vi "Get Cooler Status.vi"(8 "error in (no error)":errorcluster, 11 "Detector in":refnum<class "Detector.lvclass">) -> (0 "error out":errorcluster, 2 "Cooler status":bool, 3 "Detector out":refnum<class "Detector.lvclass">)   [LabVIEW 2015, in "Detector.lvclass"]
uses:
  Detector.lvclass
  GeneralFunctionality/GeneralFunctionality.lvclass/GeneralFunctionality.ctl
  Config/Config.lvclass
  GeneralFunctionality/GeneralFunctionality.lvclass
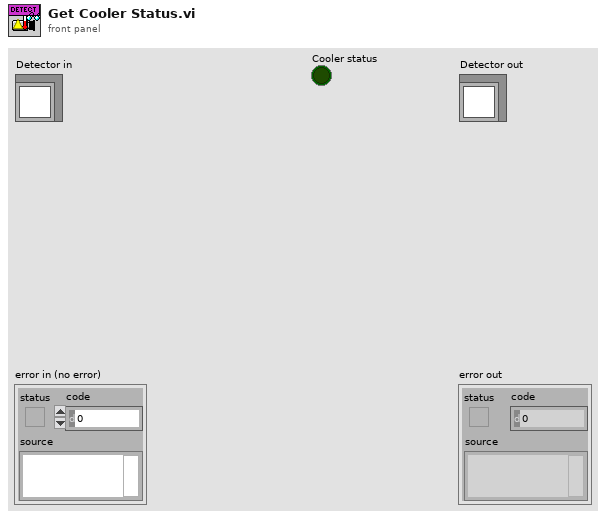
[diagram p1: front panel]
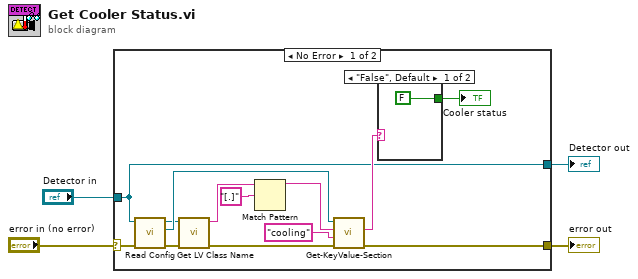
[diagram p0: block diagram]
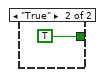
[diagram p2: hidden frame]
diagram:
  n1 = case shown="No Error" "error in (no error)" {
    selector: "error in (no error)" -> [w7 w21]
    tunnel: [w10 w21] -> w3
    tunnel: [w9 w20] -> w1
    tunnel: "Detector in" -> [w9 w20]
    frame No Error {
      n2 = call "Read Config.vi"("error in (no error)"=w7, "GeneralFunctionality en entrée"=w9) -> ("error out"=w6:errorcluster, "Config.lvclass"=w8:refnum<class "Config.lvclass">, "GeneralFunctionality en sortie"=w5:refnum<class "Detector.lvclass">)  [unwired: 7 in]
      n3 = call <vilib>:"Get LV Class Name.vi"("error in (no error)"=w6, "object"=w5) -> ("error out"=w17:errorcluster, "class name"=w16:string)  [unwired: 8 in]
      n4 = Match Pattern(string=w16, regular expression="[.]") -> (before substring=w14:string)  [unwired: 1 in, 3 out]
      n5 = call-dynamic "Get-KeyValue-Section.vi"("error in (no error)"=w17, "Key"="cooling", "Section"=w14, "Config in"=w8) -> ("error out"=w10:errorcluster, "Value"=w12:string)  [unwired: 5 in, 1 out]
      n6 = case shown="\"False\", Default" w12 {
        tunnel: [FALSE TRUE] -> w11
        frame "False", Default {
        }
        frame "True" {
        }
      }
      "Cooler status" <- w11
    }
    frame Error {
    }
  }
  "error out" <- w3
  "Detector out" <- w1
